vi "Convert Digital to Analog Waveform.vi"(6 "full scale range":dbl=10.0 format="%#_13g", 7 "channel index":i32, 9 "Number of samples":u32, 10 "Sample rate":dbl, 11 "Digital waveform in":u32[](array[numeric])) -> (1 "codes":u32[](array[numeric]), 2 "Digital waveform out":u32[](array[numeric]), 3 "Waveform":waveform(dbl))   [LabVIEW 2021]
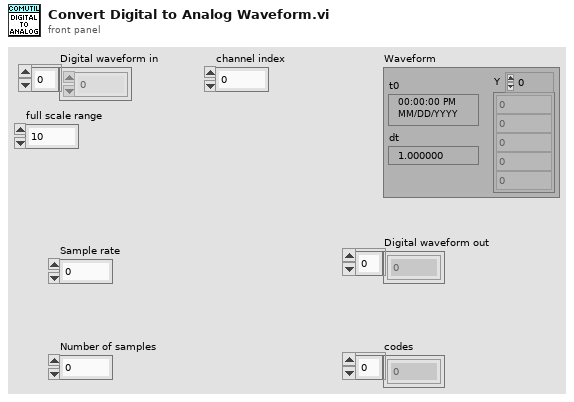
[diagram p1: front panel]
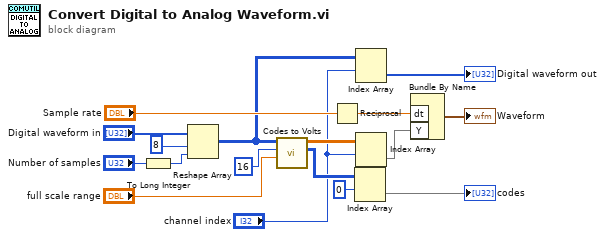
[diagram p0: block diagram]
diagram:
  n1 = To Long Integer(number="Number of samples") -> (32bit integer=w1:i32)
  n2 = Reshape Array("Digital waveform in", 8 ("dimension size"), w1) -> (w5:u32[][])
  n3 = call "Codes to Volts.vi"("full scale range"="full scale range", "number of bits"=16, "data"=w5) -> ("codes"=w8:u32[][], "scaled data"=w13:dbl[][])  [unwired: 7 in]
  n4 = Reciprocal(x="Sample rate") -> (1/x=w14:dbl)
  n5 = Index Array(array=w8, index (row)=0) -> (element=→"codes":u32[])  [unwired: 1 in]
  n6 = Index Array(array=w5, index (row)="channel index") -> (element=→"Digital waveform out":u32[])  [unwired: 1 in]
  n7 = Index Array(array=w13, index (row)="channel index") -> (element=w9:dbl[])  [unwired: 1 in]
  n8 = Bundle By Name("dt"=w14, "Y"=w9) -> (→"Waveform":waveform(dbl))  [unwired: 1 in]
